vi "get Controls Value LV.vi"(8 "error in (no error)":errorcluster, 11 "controlValsOut":dbl) -> (0 "error out":errorcluster, 3 "controlValsOut out":dbl)   [LabVIEW 2016, in "cameraLibrary.lvlib"]
doc: "Returns the current control loop values.\n\nvoid CAMERALIBRARYSHARED_EXPORT getControlsValueLV(double *controlValsOut);"
uses:
  cameraLibrary.lvlib
  cameraLibrary.dll
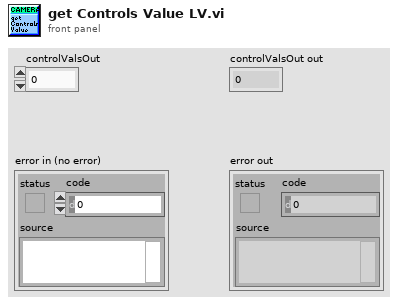
[diagram p1: front panel]
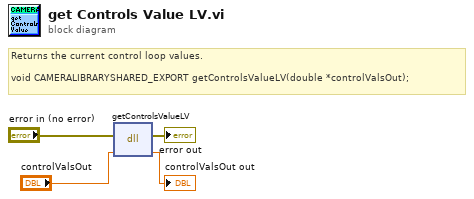
[diagram p0: block diagram]
diagram:
  # "Returns the current control loop values.\n\nvoid CAMERALIBRARYSHARED_EXPORT getControlsValueLV(double *controlValsOut);"
  n1 = dll-call lib="C:/Users/TMM/repos/EXPRES/cameraLibrary/build-cameraLibrary/labview-import/cameraLibrary.*" fn="getControlsValueLV"(error in="error in (no error)", "controlValsOut"="controlValsOut") -> (error out=→"error out":errorcluster, "controlValsOut"=→"controlValsOut out":dbl)  [unwired: 3 in, 1 out]
